vi "Handle Error.vi"(8 "error in (no error)":errorcluster, 11 "Vision in":refnum<class "Vision.lvclass">) -> (0 "error out":errorcluster, 2 "stop actor?":bool=TRUE, 3 "Vision out":refnum<class "Vision.lvclass">)   [LabVIEW 2021, in "Vision.lvlib" / "Vision.lvclass"]
doc: "(<B>Filename</B>: Actor Framework.lvlib:Actor.lvclass:Handle Error.vi)\n\nDefines how the actor handles an error that occurred while processing a message. By default, this method does nothing except stop the actor."
uses:
  Vision.lvclass
  <vilib>/ActorFramework/Actor/Actor.lvclass
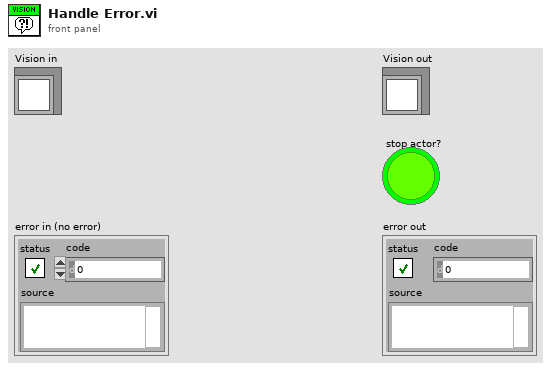
[diagram p1: front panel]
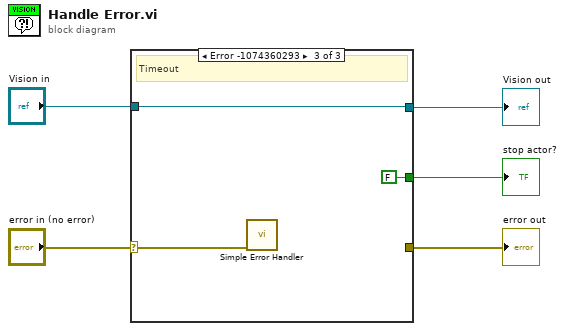
[diagram p0: block diagram]
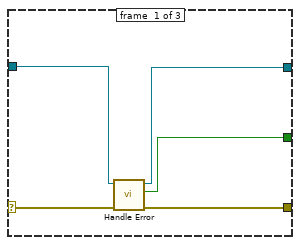
[diagram p2: hidden frame]
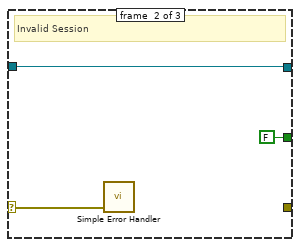
[diagram p3: hidden frame]
diagram:
  n1 = case shown="Error -1074360293" "error in (no error)" {
    selector: "error in (no error)" -> [w7 w11 w16]
    tunnel: [w10 _ _] -> w5
    tunnel: [w9 FALSE ("stop actor?") FALSE ("stop actor?")] -> w4
    tunnel: [w8 w13 w15] -> w3
    tunnel: "Vision in" -> [w6 w13 w15]
    frame #0 {
      n2 = call-parent "Handle Error.vi"("error in (no error)"=w7, "Actor in"=w6) -> ("error out"=w10:errorcluster, "stop actor?"=w9:bool, "Actor out"=w8:refnum<class "Vision.lvclass">)  [unwired: 7 in]
    }
    frame #1 {
      # "Invalid Session"
      n3 = call <vilib>:"Simple Error Handler.vi"("error in (no error)"=w11) -> ()  [unwired: 4 in, 5 out]
    }
    frame #2 {
      # "Timeout"
      n4 = call <vilib>:"Simple Error Handler.vi"("error in (no error)"=w16) -> ()  [unwired: 4 in, 5 out]
    }
  }
  "Vision out" <- w3
  "error out" <- w5
  "stop actor?" <- w4
